vi "DAC8568_setAllOutputs.vi"(3 "cameraPosition":u8, 4 "outputs 4":u32[](array[numeric]), 5 "outputs 3":u32[](array[numeric]), 6 "outputs 2":u32[](array[numeric]), 7 "location":u8, 8 "error in (no error)":errorcluster, 9 "outputs 1":u32[](array[numeric]), 10 "outputs 0":u32[](array[numeric]), 11 "reorder channels":bool) -> (0 "error out":errorcluster)   [LabVIEW 2015, in "ESLSCDLL.lvlib"]
uses:
  ESLSCDLL.lvlib
  Globals.vi
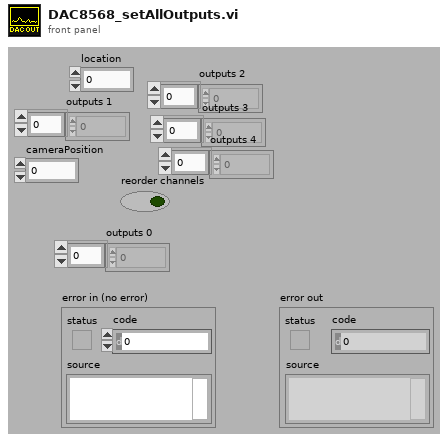
[diagram p1: front panel]
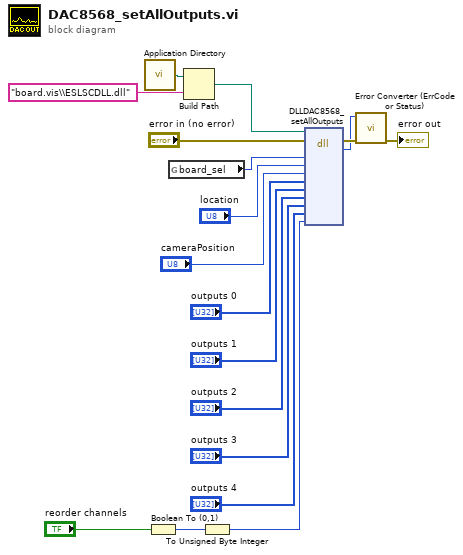
[diagram p0: block diagram]
diagram:
  n1 = call <vilib>:"Application Directory.vi"() -> ("Application Directory"=w10:path)
  n2 = Boolean To (0,1)(Boolean="reorder channels") -> (0, 1=w13:i16)
  n3 = global read "Globals.vi" "board_sel"() -> (w6:u32)
  n4 = Build Path(base path=w10, name or relative path="board.vis\\ESLSCDLL.dll") -> (appended path=w8:path)
  n5 = To Unsigned Byte Integer(number=w13) -> (unsigned 8bit integer=w11:u8)
  n6 = dll-call lib="C:/ENTW/PCIE/LV64/board.vis/ESLSCDLL.dll" fn="DLLDAC8568_setAllOutputs" ("lwlscdll.dll:DLLSetADAmpRed")(path in=w8, error in="error in (no error)", "board_sel"=w6, "location"="location", "cameraPosition"="cameraPosition", "outputs0"="outputs 0", "outputs1"="outputs 1", "outputs2"="outputs 2", "outputs3"="outputs 3", "outputs4"="outputs 4", "reorder_channel"=w11) -> (error out=w16:errorcluster, "es_status_codes"=w15:i32)  [unwired: 10 in, 1 out]
  n7 = call "Error Converter (ErrCode or Status).vi"("error in (no error)"=w16, "error code"=w15) -> ("error out"=→"error out":errorcluster)  [unwired: 9 in]
